vi "Example Pressure Control - PID Autotuning.vi"(1 "Stop":bool, 7 "Pump Controller VISA resource name":refnum<visa-resource-name>, 9 "Pump Initial Flowrate, m^3/s":dbl, 11 "Pump Pressure, bar(G)":dbl format="%#_13g", 13 "Pump PID gains":T1={"proportional gain (Kc)"=1.0, "integral time (Ti, min)"=0.0, "derivative time (Td, min)"=0.0} {"derivative time (Td, min)" format="%.3f"; "integral time (Ti, min)" format="%.3f"; "proportional gain (Kc)" format="%.3f"}) -> ()   [LabVIEW 2017]
uses:
  <vilib>/DAQmx/read.llb/DAQmx Read (Analog DBL 1Chan 1Samp).vi
  <vilib>/DAQmx/miscellaneous.llb/DAQmx Fill In Error Info.vi
  <instrlib>/Roboteq Controller KBL1xxx/Roboteq Controller KBL1xxx.lvlib
  Pump Controller.lvlib
  <vilib>/addons/control/pid/NI_PID_autopid.lvlib
panel:
  out "Measured Pressure":dbl(graph)
  out "Pump Flowrate":dbl(graph)
  out "PID output":dbl(graph)
  in  "Accept gain":bool
  out "Tuned Pump PID gains":T1={"proportional gain (Kc)"=15.221889907608013, "integral time (Ti, min)"=0.002027201803862475, "derivative time (Td, min)"=0.0002815558060920104} {"derivative time (Td, min)" format="%#.6g"; "integral time (Ti, min)" format="%#.6g"; "proportional gain (Kc)" format="%#.6g"}
  out "Tuning completed?":bool
  in  "Alpha":dbl(slide) scale=0.0..1.0
  in  "autotuning parameters":T2={"type of controller"=1, "time constant factor"=2.0, "step amplitude"=1.0} {"time constant factor" scale=0.0001..1000.0; "step amplitude" format="%.2f"; "type of controller" items=["P", "PI", "PID"]}
  in  "Reinitialize":bool
  in  "Identify and tune":bool
  in  "Initial pump parameters":T3={"process gain"=2.515490777679412, "time constant (s)"=2.529236380296785, "delay time (s)"=2.5407395402910935} {"delay time (s)" format="%.3f"; "time constant (s)" format="%.3f"; "process gain" format="%.3f"}
  in  "Automatic":bool=TRUE
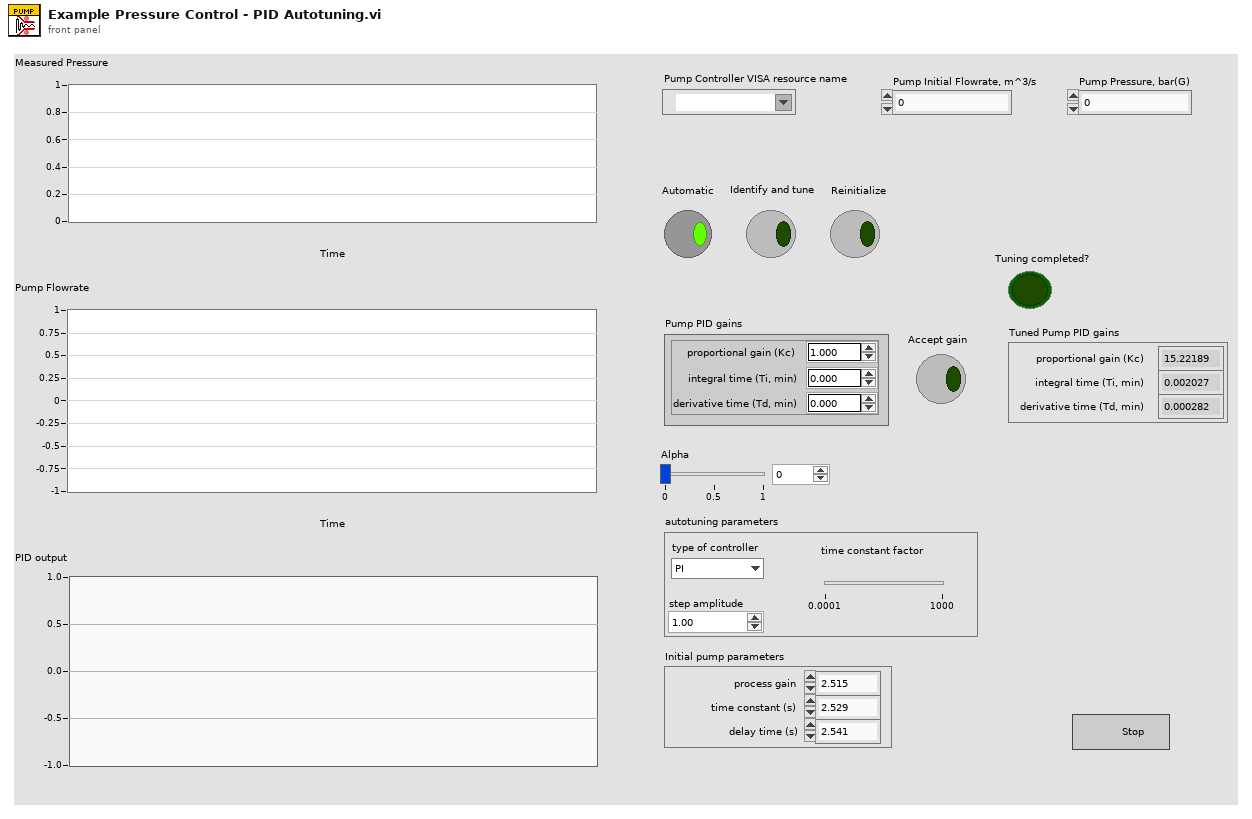
[diagram p1: front panel]
types:
  T1 = cluster{"proportional gain (Kc)":dbl, "integral time (Ti, min)":dbl, "derivative time (Td, min)":dbl}
  T2 = cluster{"type of controller":u16, "time constant factor":dbl, "step amplitude":dbl}
  T3 = cluster{"process gain":dbl, "time constant (s)":dbl, "delay time (s)":dbl}
  T4 = typedef "Roboteq Controller KBL1xxx.lvlib/Controller.ctl" = cluster{"VISA resource name out":refnum<visa-resource-name>, "MXRPM":u16}
  T5 = typedef "Pump Controller.lvlib/Pump.ctl" = cluster{"Controller":T4}
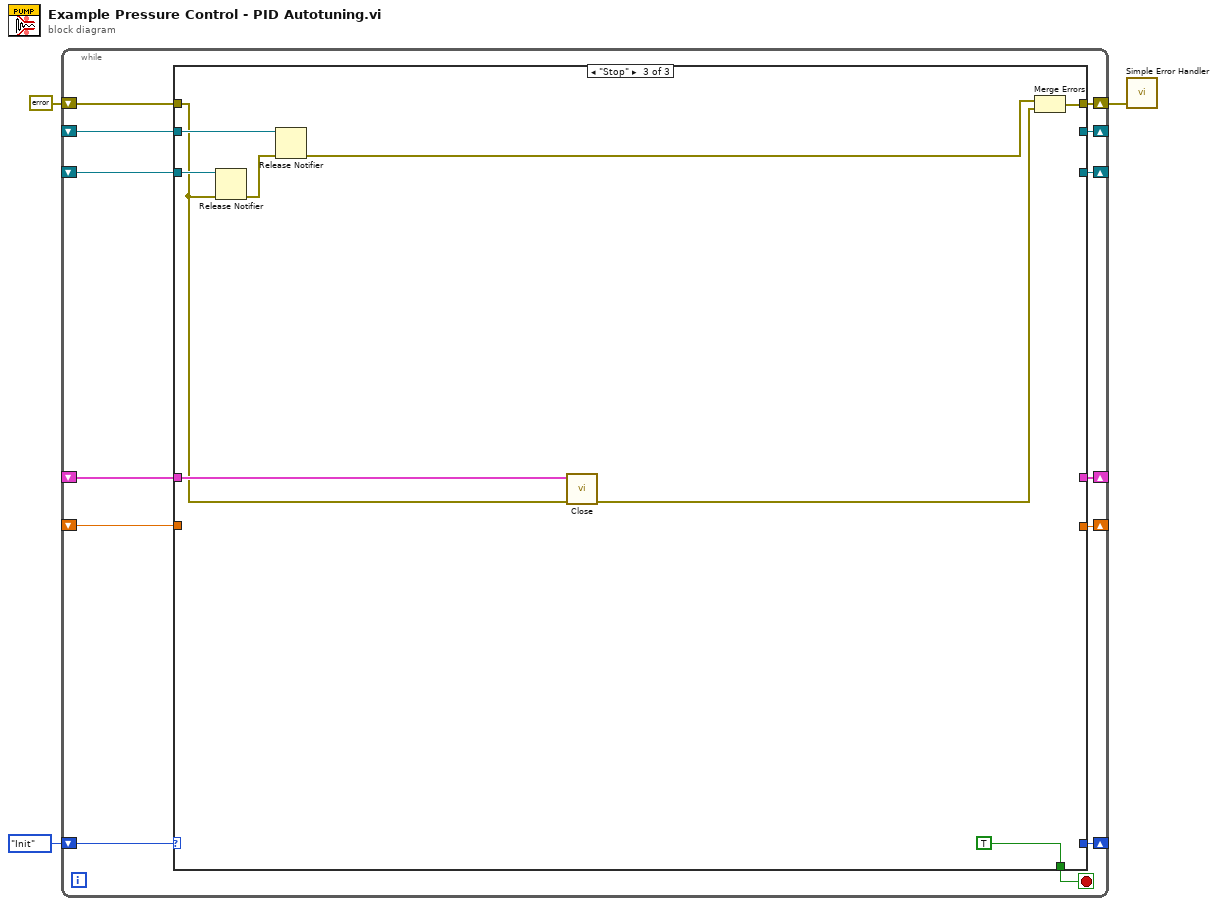
[diagram p0: block diagram]
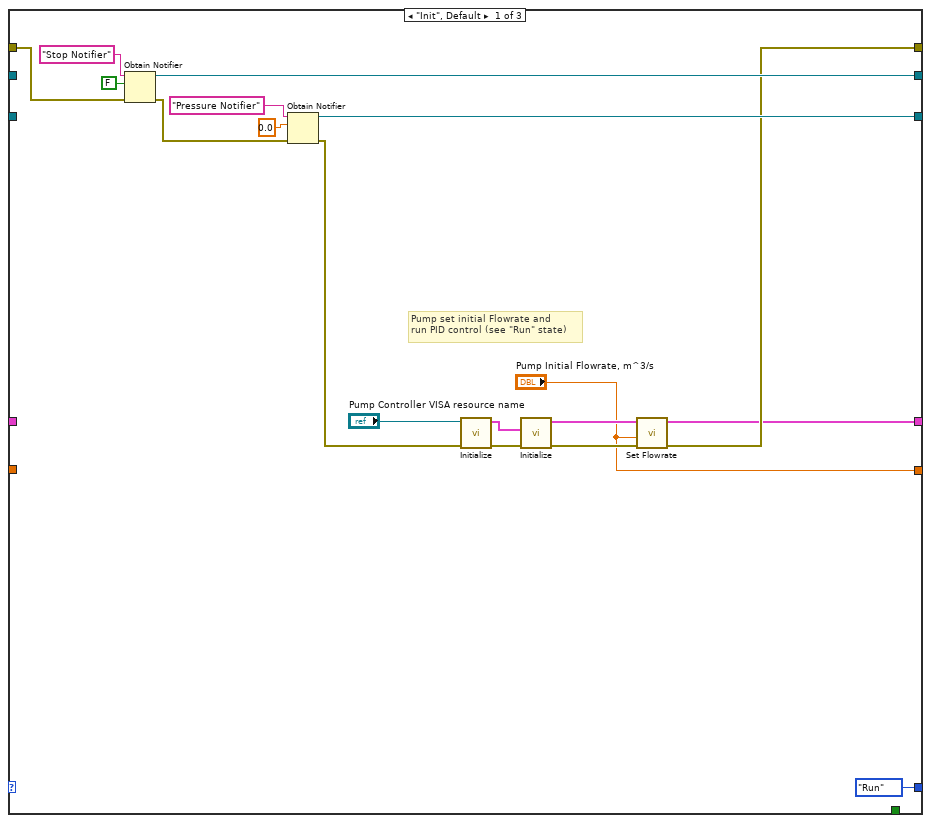
[diagram p2: hidden frame]
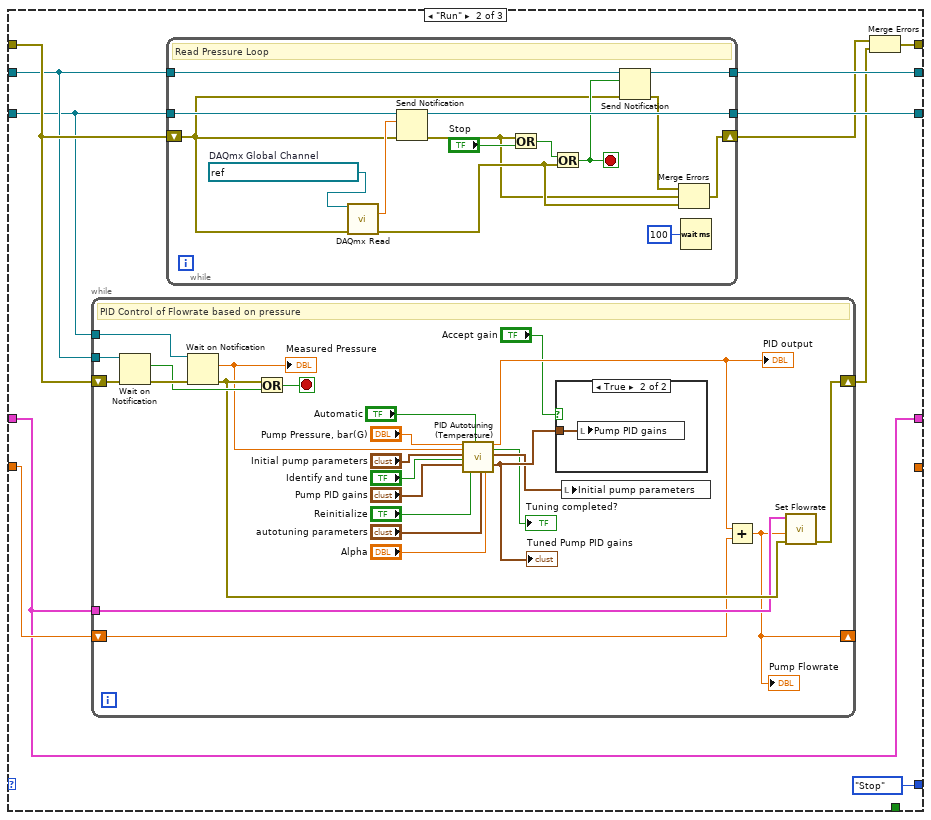
[diagram p3: hidden frame]
diagram:
  n1 = while {
    shift-right: [w15] -> _
    shift-left: enum16{"Init", "Run", "Stop"}."Init" ("State") -> [w16]
    shift-right: [w13] -> _
    shift-left: _ -> [w10]
    shift-right: [w12] -> _
    shift-left: _ -> [w9]
    shift-right: [w8] -> w1
    shift-left: errorcluster {"status"=FALSE, "code"=0, "source"=""} ("error IO") -> [w11]
    shift-right: [w7] -> _
    shift-left: _ -> [w6]
    shift-right: [w5] -> _
    shift-left: _ -> [w4]
    stop <- w14 stop-if-true
    n2 = case shown="\"Stop\"" w16 {
      tunnel: [enum16{"Init", "Run", "Stop"}."Run" ("State") enum16{"Init", "Run", "Stop"}."Stop" ("State") _] -> w15
      tunnel: [_ _ TRUE] -> w14
      tunnel: [w28 w43 _] -> w13
      tunnel: [w27 w42 _] -> w12
      tunnel: w11 -> [w25 w44 w88]
      tunnel: w10 -> [_ w41 w92]
      tunnel: w9 -> [_ w40 w93]
      tunnel: [w20 w39 w90] -> w8
      tunnel: [w19 w35 _] -> w7
      tunnel: w6 -> [_ w35 w91]
      tunnel: ["Pump Initial Flowrate, m^3/s" _ _] -> w5
      tunnel: w4 -> [_ w36 _]
      frame "Init", Default {
        # "Pump set initial Flowrate and \nrun PID control (see \"Run\" state)"
        n3 = Obtain Notifier(name (unnamed)="Stop Notifier", notification data type=FALSE, error in (no error)=w25) -> (notifier out=w28:refnum<notifier>, error out=w33:errorcluster)  [unwired: 1 in, 1 out]
        n4 = Obtain Notifier(name (unnamed)="Pressure Notifier", notification data type=0.0, error in (no error)=w33) -> (notifier out=w27:refnum<notifier>, error out=w17:errorcluster)  [unwired: 1 in, 1 out]
        n5 = call <instrlib>:"Initialize.vi"("error in (no error)"=w17, "VISA resource name"="Pump Controller VISA resource name") -> ("error out"=w24:errorcluster, "Controller"=w23:T4)  [unwired: 8 in]
        n6 = call <instrlib>:"Initialize.vi"("error in (no error)"=w24, "Controller"=w23) -> ("error out"=w22:errorcluster, "Pump"=w21:T5)  [unwired: 8 in]
        n7 = call "Set Flowrate.vi"("error in (no error)"=w22, "Flowrate, m^3/s"="Pump Initial Flowrate, m^3/s", "Pump in"=w21) -> ("error out"=w20:errorcluster, "Pump out"=w19:T5)  [unwired: 7 in]
      }
      frame "Run" {
        n8 = while {
          tunnel: w41 -> [w69]
          tunnel: w40 -> [w67]
          shift-right: [w63] -> w37
          shift-left: w44 -> [w70]
          shift-right: [w46] -> _
          shift-left: w36 -> [w52]
          tunnel: w35 -> [w62]
          stop <- w65 stop-if-true
          # "PID Control of Flowrate based on pressure"
          n9 = Wait on Notification(notifier=w69, error in (no error)=w70) -> (notification=w66:bool, error out=w68:errorcluster)  [unwired: 2 in, 2 out]
          n10 = Wait on Notification(notifier=w67, error in (no error)=w68) -> (notification=w60:dbl, error out=w64:errorcluster)  [unwired: 2 in, 2 out]
          "Measured Pressure" <- w60
          n11 = Or(x=w64, y=w66) -> (x .or. y?=w65:bool)
          n12 = call <vilib>:"PID Autotuning (Temperature).vi"("desired temperature"="Pump Pressure, bar(G)", "measured temperature"=w60, "plant parameters in"="Initial pump parameters", "autotune? (F)"="Identify and tune", "PID gains in"="Pump PID gains", "reinitialize? (F)"="Reinitialize", "auto? (T)"="Automatic", "autotuning parameters"="autotuning parameters", "alpha"="Alpha") -> ("output"=w51:dbl, "tuning completed?"=→"Tuning completed?":bool, "plant parameters out"=w48:T3, "PID gains out"=w49:T1)  [unwired: 7 in]
          "PID output" <- w51
          "Tuned Pump PID gains" <- w49
          n13 = case shown="True" "Accept gain" {
            tunnel: w49 -> [_ w71]
            frame False {
            }
            frame True {
              n14 = local write "Pump PID gains"(w71) -> ()
            }
          }
          n15 = local write "Initial pump parameters"(w48) -> ()
          n16 = Add(x=w51, y=w52) -> (x+y=w46:dbl)
          "Pump Flowrate" <- w46
          n17 = call "Set Flowrate.vi"("error in (no error)"=w64, "Flowrate, m^3/s"=w46, "Pump in"=w62) -> ("error out"=w63:errorcluster)  [unwired: 7 in, 1 out]
        }
        n18 = while {
          tunnel: w41 -> [w85]
          tunnel: [w84] -> w43
          tunnel: w40 -> [w83]
          tunnel: [w82] -> w42
          shift-right: [w75] -> w38
          shift-left: w44 -> [w74]
          stop <- w76 stop-if-true
          w72 = refnum<k21> "PressureVirtualChannel"  # DAQmx Global Channel
          # "Read Pressure Loop"
          n19 = call-poly <vilib>:"DAQmx Read.vi"("task/channels in"=w72, "error in"=w74) -> ("data"=w80:dbl, "error out"=w78:errorcluster)  [unwired: 11 in, 1 out]
          n20 = Send Notification(notification=w80, notifier=w83, error in (no error)=w74) -> (notifier out=w82:refnum<notifier>, error out=w77:errorcluster)
          n21 = Or(x=w77, y="Stop") -> (x .or. y?=w79:bool)
          n22 = Or(x=w79, y=w78) -> (x .or. y?=w76:bool)
          n23 = Send Notification(notification=w76, notifier=w85, error in (no error)=w74) -> (notifier out=w84:refnum<notifier>, error out=w73:errorcluster)
          n24 = Merge Errors(w73, w77, w78) -> (w75:errorcluster)
          n25 = Wait (ms)(milliseconds to wait=u32 100) -> ()  [unwired: 1 out]
        }
        n26 = Merge Errors(w38, w37) -> (w39:errorcluster)
      }
      frame "Stop" {
        n27 = Release Notifier(notifier=w93, error in (no error)=w88) -> (error out=w94:errorcluster)  [unwired: 1 in, 2 out]
        n28 = Release Notifier(notifier=w92, error in (no error)=w94) -> (error out=w89:errorcluster)  [unwired: 1 in, 2 out]
        n29 = call "Close.vi"("error in (no error)"=w88, "Pump in"=w91) -> ("error out"=w87:errorcluster)  [unwired: 9 in]
        n30 = Merge Errors(w89, w87) -> (w90:errorcluster)
      }
    }
  }
  n31 = call <vilib>:"Simple Error Handler.vi"("error in (no error)"=w1) -> ()  [unwired: 4 in, 5 out]
